vi "Configure Ossiloscope Settings.vi"(8 "error in":errorcluster, 10 "input settings":T1={"LeCroy IP"="169.254.20.90", "Ch1"={"On/Off"=FALSE, "Bandwidth (Dropdown)"=0, "Vertical Range (V)"=5000.0, "Vertical Offset (V)"=0.0}, "Ch2"={"On/Off"=FALSE, "Bandwidth (Dropdown)"=0, "Vertical Range (V)"=0.2, "Vertical Offset (V)"=0.0}, "Ch3"={"On/Off"=TRUE, "Bandwidth (Dropdown)"=0, "Vertical Range (V)"=1.2, "Vertical Offset (V)"=0.0}, "Ch4"={"On/Off"=TRUE, "Bandwidth (Dropdown)"=0, "Vertical Range (V)"=0.2, "Vertical Offset (V)"=0.0}, "T axis"={"Time base (s/div)"=0.0002, "Time offset (s)"=0.0, "Max Sample Points"=0}, "Trig"={"Trigger mode"=2, "Trigger Slope"=0, "Trigger Source"=1, "Trigger Level (V)"=0.04}, "Timeout (ms)"=0.0} caption="Settings" {"Trig"."Trigger mode" items=["Auto", "Normal", "Single", "Single, auto trigger"]; "Trig"."Trigger Slope" items=["Rising", "Falling"]; "Trig"."Trigger Source" items=["Channel 1", "Channel 2", "Channel 3", "Channel 4", "External", "Power Line"]; "Trig"."Trigger Level (V)" format="%#_6p"; "T axis"."Max Sample Points" format="%.0p" items=["50"=50, "100"=100, "250"=250, "500"=500, "1000"=1000, "2500"=2500, "5K"=5000, "10K"=10000, "25K"=25000, "50K"=50000, "100K"=100000, "250K"=250000, "500K"=500000, "1M"=1000000, "2M"=2000000, "2.5M"=2500000, "5M"=5000000, "10M"=10000000, "25M"=25000000, "50M"=50000000, "100M"=100000000]; "T axis"."Time base (s/div)" format="%#_6p"; "Ch4"."Bandwidth (Dropdown)" items=["Full", "20MHZ", "25MHZ", "200MHZ", "250MHZ", "1GHZ", "3GHZ", "4GHZ"]; "Ch3"."Bandwidth (Dropdown)" items=["Full", "20MHZ", "25MHZ", "200MHZ", "250MHZ", "1GHZ", "3GHZ", "4GHZ"]; "Ch2"."Bandwidth (Dropdown)" items=["Full", "20MHZ", "25MHZ", "200MHZ", "250MHZ", "1GHZ", "3GHZ", "4GHZ"]; "Ch1"."Bandwidth (Dropdown)" items=["Full", "20MHZ", "25MHZ", "200MHZ", "250MHZ", "1GHZ", "3GHZ", "4GHZ"]}, 11 "VISA resource name in":refnum<visa-resource-name>) -> (0 "error out":errorcluster, 1 "Channels to read out":i32[](array[numeric]), 2 "output settings":T1={"LeCroy IP"="169.254.20.90", "Ch1"={"On/Off"=FALSE, "Bandwidth (Dropdown)"=0, "Vertical Range (V)"=5000.0, "Vertical Offset (V)"=0.0}, "Ch2"={"On/Off"=FALSE, "Bandwidth (Dropdown)"=0, "Vertical Range (V)"=0.2, "Vertical Offset (V)"=0.0}, "Ch3"={"On/Off"=TRUE, "Bandwidth (Dropdown)"=0, "Vertical Range (V)"=1.2, "Vertical Offset (V)"=0.0}, "Ch4"={"On/Off"=TRUE, "Bandwidth (Dropdown)"=0, "Vertical Range (V)"=0.2, "Vertical Offset (V)"=0.0}, "T axis"={"Time base (s/div)"=0.0002, "Time offset (s)"=0.0, "Max Sample Points"=0}, "Trig"={"Trigger mode"=2, "Trigger Slope"=0, "Trigger Source"=1, "Trigger Level (V)"=0.04}, "Timeout (ms)"=0.0} caption="Settings" {"Trig"."Trigger mode" items=["Auto", "Normal", "Single", "Single, auto trigger"]; "Trig"."Trigger Slope" items=["Rising", "Falling"]; "Trig"."Trigger Source" items=["Channel 1", "Channel 2", "Channel 3", "Channel 4", "External", "Power Line"]; "Trig"."Trigger Level (V)" format="%#_6p"; "T axis"."Max Sample Points" format="%.0p" items=["50"=50, "100"=100, "250"=250, "500"=500, "1000"=1000, "2500"=2500, "5K"=5000, "10K"=10000, "25K"=25000, "50K"=50000, "100K"=100000, "250K"=250000, "500K"=500000, "1M"=1000000, "2M"=2000000, "2.5M"=2500000, "5M"=5000000, "10M"=10000000, "25M"=25000000, "50M"=50000000, "100M"=100000000]; "T axis"."Time base (s/div)" format="%#_6p"; "Ch4"."Bandwidth (Dropdown)" items=["Full", "20MHZ", "25MHZ", "200MHZ", "250MHZ", "1GHZ", "3GHZ", "4GHZ"]; "Ch3"."Bandwidth (Dropdown)" items=["Full", "20MHZ", "25MHZ", "200MHZ", "250MHZ", "1GHZ", "3GHZ", "4GHZ"]; "Ch2"."Bandwidth (Dropdown)" items=["Full", "20MHZ", "25MHZ", "200MHZ", "250MHZ", "1GHZ", "3GHZ", "4GHZ"]; "Ch1"."Bandwidth (Dropdown)" items=["Full", "20MHZ", "25MHZ", "200MHZ", "250MHZ", "1GHZ", "3GHZ", "4GHZ"]}, 3 "VISA resource name out":refnum<visa-resource-name>)   [LabVIEW 2013]
uses:
  Settings_TypeDef.ctl
  <instrlib>/LeCroy Wave Series/Public/Configure/Configure Edge Trigger.vi
  <instrlib>/LeCroy Wave Series/LeCroy Wave Series.lvlib
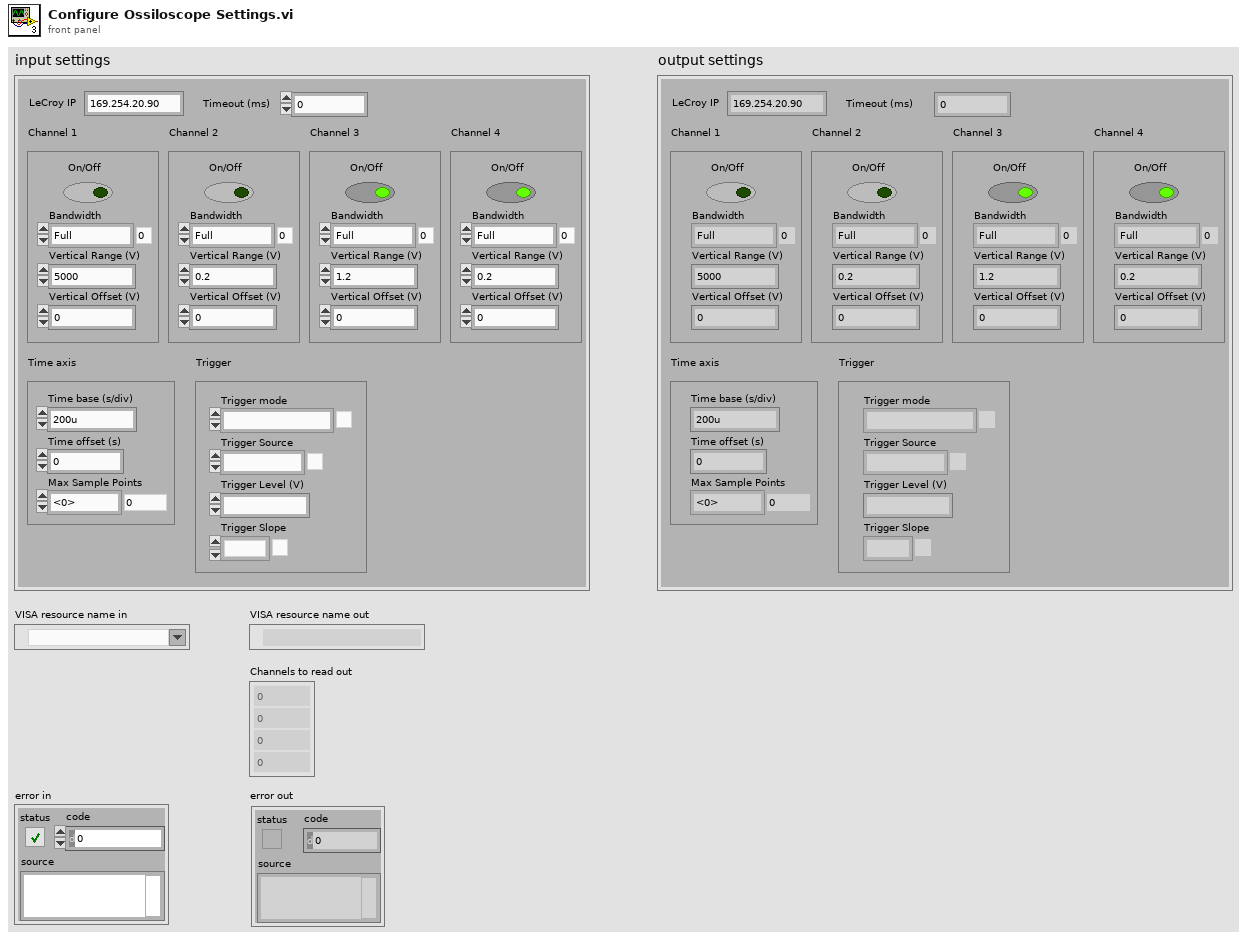
[diagram p1: front panel]
types:
  T1 = typedef "Settings_TypeDef.ctl" = cluster{"LeCroy IP":string, "Ch1":cluster{"On/Off":bool, "Bandwidth (Dropdown)":u16, "Vertical Range (V)":dbl, "Vertical Offset (V)":dbl}, "Ch2":cluster{"On/Off":bool, "Bandwidth (Dropdown)":u16, "Vertical Range (V)":dbl, "Vertical Offset (V)":dbl}, "Ch3":cluster{"On/Off":bool, "Bandwidth (Dropdown)":u16, "Vertical Range (V)":dbl, "Vertical Offset (V)":dbl}, "Ch4":cluster{"On/Off":bool, "Bandwidth (Dropdown)":u16, "Vertical Range (V)":dbl, "Vertical Offset (V)":dbl}, "T axis":cluster{"Time base (s/div)":dbl, "Time offset (s)":dbl, "Max Sample Points":i32}, "Trig":cluster{"Trigger mode":u16, "Trigger Slope":u16, "Trigger Source":u16, "Trigger Level (V)":dbl}, "Timeout (ms)":dbl}
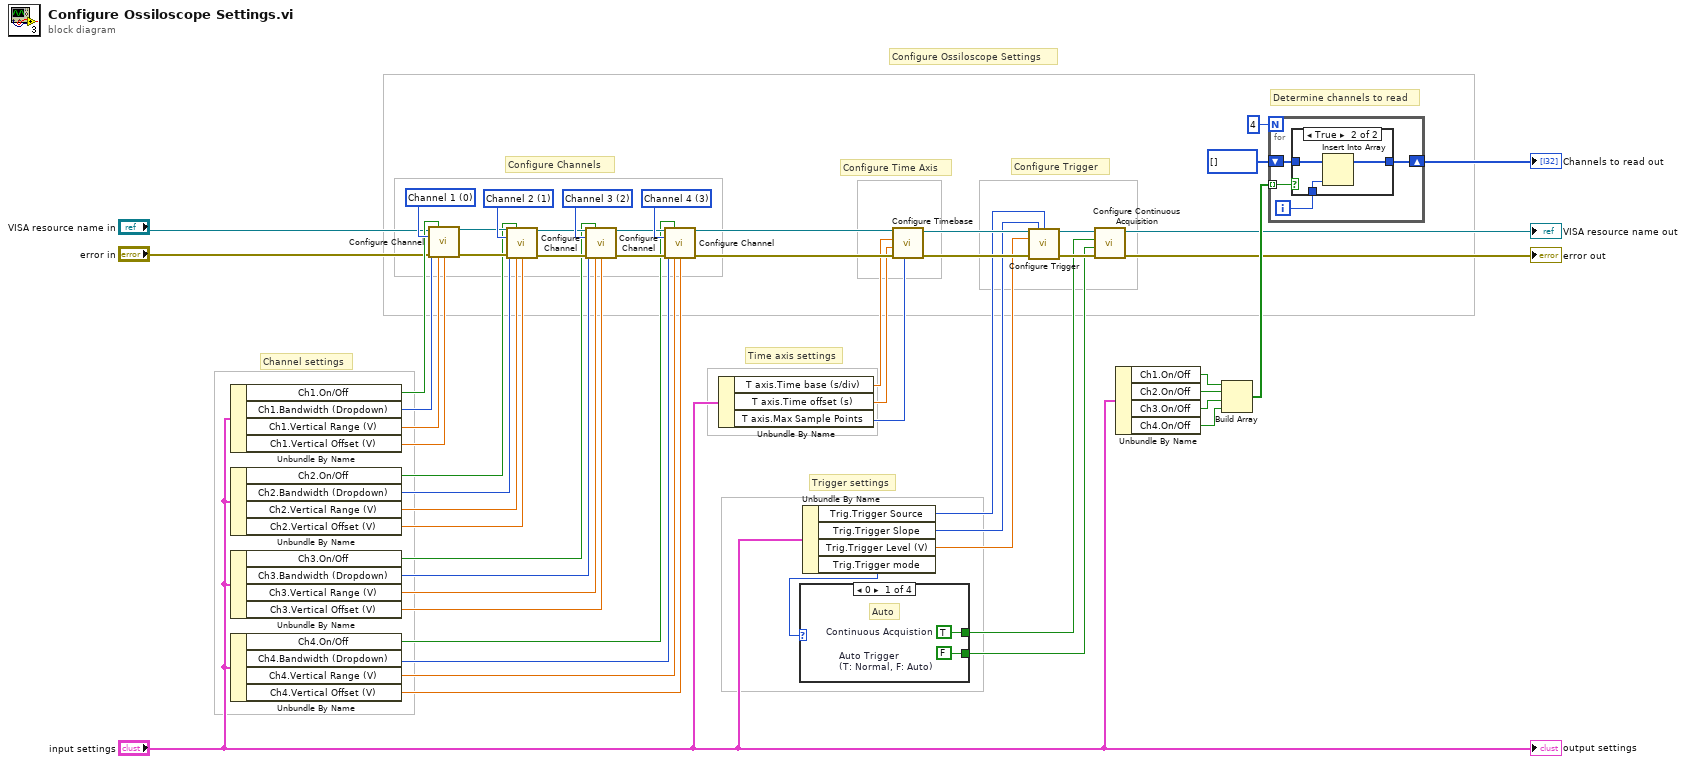
[diagram p0: block diagram]
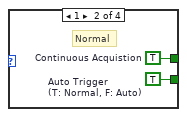
[diagram p3: hidden frame]
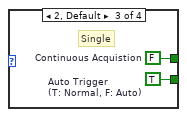
[diagram p4: hidden frame]
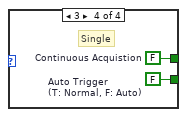
[diagram p5: hidden frame]
diagram:
  w51 = u16 3 items=["Channel 1", "Channel 2", "Channel 3", "Channel 4"] ("Source (0: Channel 1)")
  w52 = u16 2 items=["Channel 1", "Channel 2", "Channel 3", "Channel 4"] ("Source (0: Channel 1)")
  w53 = u16 1 items=["Channel 1", "Channel 2", "Channel 3", "Channel 4"] ("Source (0: Channel 1)")
  w54 = u16 0 items=["Channel 1", "Channel 2", "Channel 3", "Channel 4"] ("Source (0: Channel 1)")
  # "Determine channels to read"
  # "Trigger settings"
  # "Configure Trigger"
  # "Configure Time Axis"
  # "Time axis settings"
  # "Channel settings"
  # "Configure Channels"
  # "Configure Ossiloscope Settings"
  n1 = Unbundle By Name("input settings") -> ("Ch1.On/Off"=w32:bool, "Ch1.Bandwidth (Dropdown)"=w37:u16, "Ch1.Vertical Range (V)"=w38:dbl, "Ch1.Vertical Offset (V)"=w39:dbl)
  n2 = Unbundle By Name("input settings") -> ("Ch2.On/Off"=w29:bool, "Ch2.Bandwidth (Dropdown)"=w30:u16, "Ch2.Vertical Range (V)"=w31:dbl, "Ch2.Vertical Offset (V)"=w28:dbl)
  n3 = Unbundle By Name("input settings") -> ("Ch3.On/Off"=w23:bool, "Ch3.Bandwidth (Dropdown)"=w22:u16, "Ch3.Vertical Range (V)"=w21:dbl, "Ch3.Vertical Offset (V)"=w20:dbl)
  n4 = Unbundle By Name("input settings") -> ("Ch4.On/Off"=w25:bool, "Ch4.Bandwidth (Dropdown)"=w26:u16, "Ch4.Vertical Range (V)"=w27:dbl, "Ch4.Vertical Offset (V)"=w24:dbl)
  n5 = call <instrlib>:"Configure Channel.vi"("VISA resource name"="VISA resource name in", "Enable Channel (T:On)"=w32, "Bandwidth (0: Full)"=w37, "Channel (0: Channel 1)"=w54, "error in (no error)"="error in", "Vertical Range (10.0 V)"=w38, "Vertical Offset (0.0 V)"=w39) -> ("VISA resource name out"=w50:refnum<visa-resource-name>, "error out"=w49:errorcluster)  [unwired: 7 in]
  n6 = call <instrlib>:"Configure Channel.vi"("VISA resource name"=w50, "Enable Channel (T:On)"=w29, "Bandwidth (0: Full)"=w30, "Channel (0: Channel 1)"=w53, "error in (no error)"=w49, "Vertical Range (10.0 V)"=w31, "Vertical Offset (0.0 V)"=w28) -> ("VISA resource name out"=w47:refnum<visa-resource-name>, "error out"=w48:errorcluster)  [unwired: 7 in]
  n7 = call <instrlib>:"Configure Channel.vi"("VISA resource name"=w47, "Enable Channel (T:On)"=w23, "Bandwidth (0: Full)"=w22, "Channel (0: Channel 1)"=w52, "error in (no error)"=w48, "Vertical Range (10.0 V)"=w21, "Vertical Offset (0.0 V)"=w20) -> ("VISA resource name out"=w46:refnum<visa-resource-name>, "error out"=w45:errorcluster)  [unwired: 7 in]
  n8 = call <instrlib>:"Configure Channel.vi"("VISA resource name"=w46, "Enable Channel (T:On)"=w25, "Bandwidth (0: Full)"=w26, "Channel (0: Channel 1)"=w51, "error in (no error)"=w45, "Vertical Range (10.0 V)"=w27, "Vertical Offset (0.0 V)"=w24) -> ("VISA resource name out"=w44:refnum<visa-resource-name>, "error out"=w43:errorcluster)  [unwired: 7 in]
  n9 = Unbundle By Name("input settings") -> ("T axis.Time base (s/div)"=w19:dbl, "T axis.Time offset (s)"=w18:dbl, "T axis.Max Sample Points"=w17:i32)
  n10 = Unbundle By Name("input settings") -> ("Trig.Trigger Source"=w10:u16, "Trig.Trigger Slope"=w9:u16, "Trig.Trigger Level (V)"=w8:dbl, "Trig.Trigger mode"=w7:u16)
  n11 = case shown="0" w7 {
    tunnel: [w56 w58 w60 w62] -> w11
    tunnel: [w55 w57 w59 w61] -> w12
    frame 0 {
      w55 = FALSE  # Auto Trigger (T: Normal, F: Auto)
      w56 = TRUE  # Continuous Acquistion
      # "Auto"
    }
    frame 1 {
      w57 = TRUE  # Auto Trigger (T: Normal, F: Auto)
      w58 = TRUE  # Continuous Acquistion
      # "Normal"
    }
    frame 2, Default {
      w59 = TRUE  # Auto Trigger (T: Normal, F: Auto)
      w60 = FALSE  # Continuous Acquistion
      # "Single"
    }
    frame 3 {
      w61 = FALSE  # Auto Trigger (T: Normal, F: Auto)
      w62 = FALSE  # Continuous Acquistion
      # "Single"
    }
  }
  n12 = call <instrlib>:"Configure Timebase.vi"("Maximum Sample Points (500)"=w17, "error in (no error)"=w43, "Position (0.0 s)"=w18, "Timebase (0.0005 s)"=w19, "VISA resource name"=w44) -> ("error out"=w13:errorcluster, "VISA resource name out"=w16:refnum<visa-resource-name>)  [unwired: 5 in]
  n13 = call-poly <instrlib>:"Configure Trigger.vi"("VISA resource name"=w16, "Trigger Slope (0: Rising)"=w9, "Trigger Source (0: Channel 1)"=w10, "Trigger Level (0.0 V)"=w8, "error in (no error)"=w13) -> ("VISA resource name out"=w15:refnum<visa-resource-name>, "error out"=w14:errorcluster)  [unwired: 9 in]
  n14 = call <instrlib>:"Configure Continuous Acquisition.vi"("error in (no error)"=w14, "Auto Trigger Enabled (T: Normal)"=w12, "Continuous Acquisition Mode (T: On)"=w11, "VISA resource name"=w15) -> ("error out"=→"error out":errorcluster, "VISA resource name out"=→"VISA resource name out":refnum<visa-resource-name>)  [unwired: 6 in]
  n15 = Unbundle By Name("input settings") -> ("Ch1.On/Off"=w36:bool, "Ch2.On/Off"=w35:bool, "Ch3.On/Off"=w34:bool, "Ch4.On/Off"=w33:bool)
  n16 = Build Array(w36, w35, w34, w33) -> (w42:bool[])
  n17 = for {
    N: 4 -> [_]
    tunnel: w42 -> [w63] mode=indexing
    shift-right: [w64] -> w1
    shift-left: i32[] [] -> [w65]
    i -> [w66]
    n18 = case shown="True" w63 {
      tunnel: w66 -> [_ w70]
      tunnel: w65 -> [w67 w69]
      tunnel: [w67 w68] -> w64
      frame False {
      }
      frame True {
        n19 = Insert Into Array(array=w69, new element=w70) -> (w68:i32[])  [unwired: 1 in]
      }
    }
  }
  "Channels to read out" <- w1
  "output settings" <- "input settings"
